vi "Flush.vi"(11 "TypedCircularBuffer in":refnum<class "VarCircularBuffer.lvclass">) -> (2 "Flushed Buffer":variant[](array[variant]), 3 "TypedCircularBuffer out":refnum<class "VarCircularBuffer.lvclass">)   [LabVIEW 2024, in "VarCircularBuffer.lvclass"]
uses:
  VarCircularBuffer.lvclass
  VarCircularBuffer.lvclass/VarCircularBuffer.ctl
  9e5e380d-a9b6-4c49-a1d6-4829efd6953e.vi
  9e5e380d-a9b6-4c49-a1d6-4829efd6953e.vi/83cdeaba-e1ff-493a-b62c-1f93efcfb5e6.vi
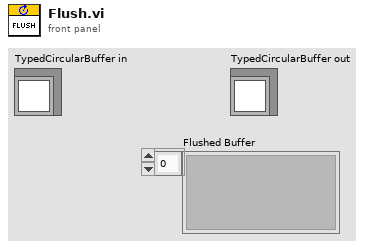
[diagram p1: front panel]
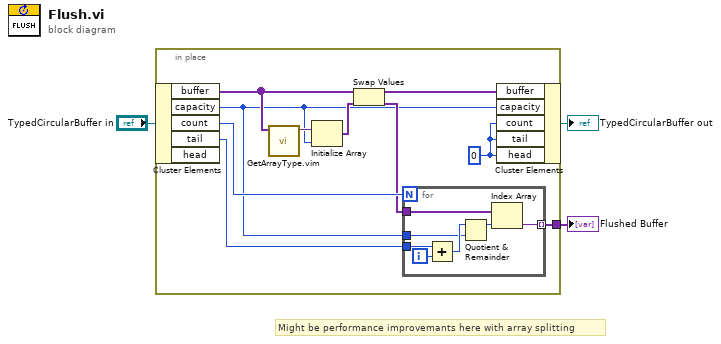
[diagram p0: block diagram]
diagram:
  # "Might be performance improvemants here with array splitting"
  n1 = in-place {
    in-place-border: [w12] -> w1
    w9 = u32 0 ("head")
    n2 = in-place-cluster #1("TypedCircularBuffer in") -> ("buffer"=w8:variant[], "capacity"=w4:u32, "count"=w11:u32, "tail"=w10:u32)  [unwired: 1 out]
    n3 = call "GetArrayType.vim"("buffer"=w8) -> ("Placeholder Type"=w13:variant)  [unwired: 10 in]
    n4 = Initialize Array(w13, w4) -> (w7:variant[])
    n5 = Swap Values(12:w8, 14:w7) -> (1:w5:variant[], 3:w6:variant[])  [unwired: 1 in]
    n6 = for {
      N: w11 -> [_]
      tunnel: w6 -> [w20]
      tunnel: w10 -> [w18]
      tunnel: w4 -> [w15]
      tunnel: [w14] -> w12 mode=indexing
      i -> [w19]
      n7 = Add(x=w18, y=w19) -> (x+y=w17:u32)
      n8 = Quotient & Remainder(x=w17, y=w15) -> (x-y*floor(x/y)=w16:u32)  [unwired: 1 out]
      n9 = Index Array(array=w20, index=w16) -> (element=w14:variant)
    }
    n10 = in-place-cluster #1("buffer"=w5, "capacity"=w4, "count"=w9, "tail"=w9, "head"=w9) -> (→"TypedCircularBuffer out":refnum<class "VarCircularBuffer.lvclass">)
  }
  "Flushed Buffer" <- w1
